vi "Plot legend tester.vi"() -> ()   [LabVIEW 2020]
uses:
  XGrapher.xctl
  Typedefs/Xctrl-ROI type enum.ctl
  Typedefs/Xctl-XY data type definition.ctl
  Typedefs/Xcrtl-Data format definition.ctl
  Typedefs/Xctrl-Data array.ctl
  Data 1.ctl
panel:
  in  "Data In":T1
  out "XY Graph":T6(graph)
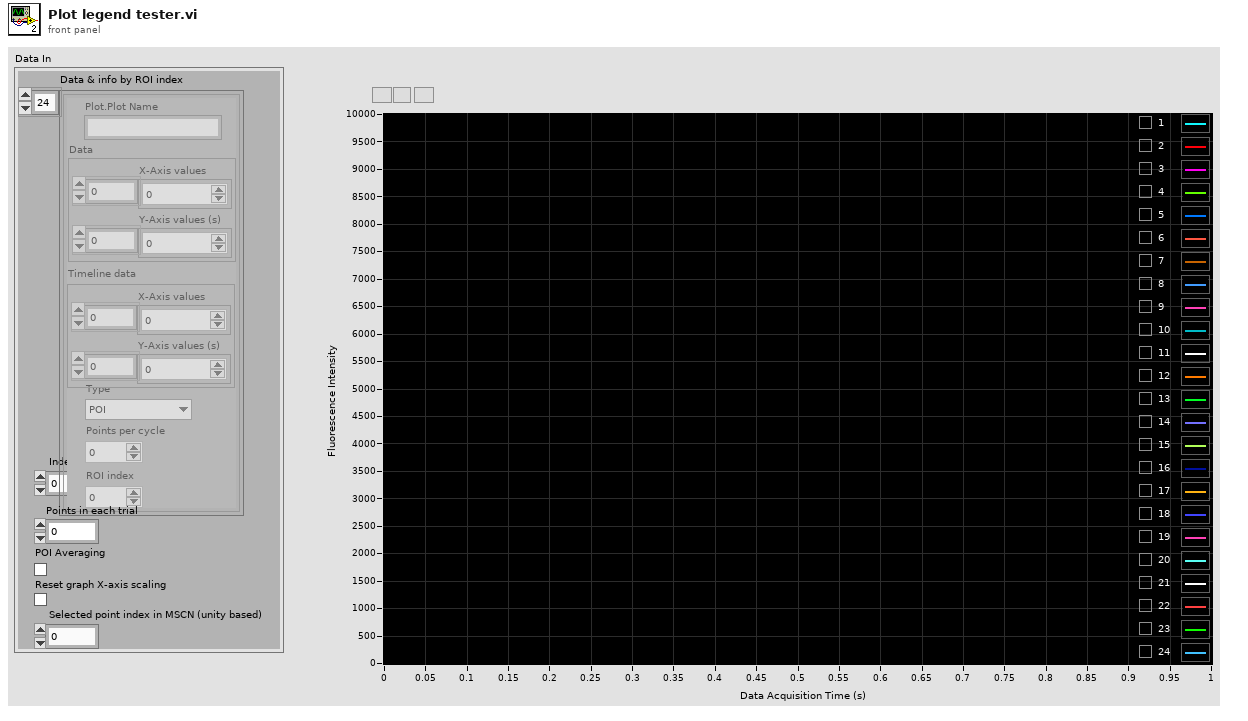
[diagram p1: front panel]
types:
  T1 = typedef "XGrapher.xctl/Data 1.ctl" = cluster{"Data & info by ROI index":T2, "Index of selected plot":u16, "Points in each trial":i32, "POI Averaging":bool, "Reset graph X-axis scaling":bool, "Selected point index in MSCN (unity based)":u16}
  T2 = typedef "Xctrl-Data array.ctl" = T3[]
  T3 = typedef "XGrapher.xctl/Xcrtl-Data format definition.ctl" = cluster{"Plot.Plot Name":string, "Data":T4, "Timeline data":T4, "Type":T5, "Points per cycle":u16, "ROI index":u16}
  T4 = typedef "XGrapher.xctl/Xctl-XY data type definition.ctl" = cluster{"X-Axis values":sgl[], "Y-Axis values (s)":sgl[]}
  T5 = typedef "Xctrl-ROI type enum.ctl" = enum16{"POI", "Mini-scan", "Group"}
  T6 = cluster{"X-Axis values":dbl[], "Y-Axis values":dbl[]}[]
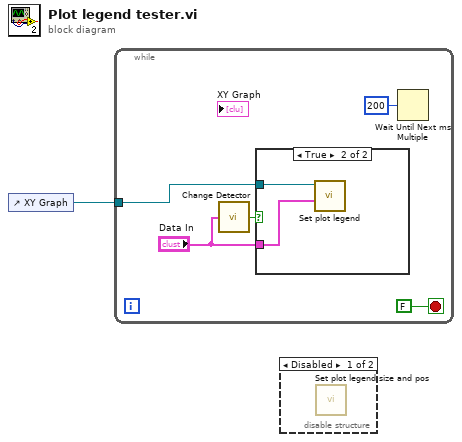
[diagram p0: block diagram]
diagram:
  n1 = control-ref of="XY Graph"() -> (w1:refnum<vi>)
  n2 = while {
    tunnel: w1 -> [w6]
    stop <- FALSE stop-if-true
    n3 = call <userlib>:"Change Detector.vi"("Value"="Data In") -> ("Changed?"=w2:bool)
    n4 = case shown="True" w2 {
      tunnel: w6 -> [_ w8]
      tunnel: "Data In" -> [_ w7]
      frame False {
      }
      frame True {
        n5 = call "Set plot legend.vi"("Data In"=w7, "XYGraph in"=w8) -> ()  [unwired: 8 in, 2 out]
      }
    }
    n6 = Wait Until Next ms Multiple(millisecond multiple=u32 200) -> ()  [unwired: 1 out]
  }
  n7 = disable-structure shown="Disabled" {
    frame Disabled {
      n8 = call "Set plot legend size and pos.vi"() -> ()  [unwired: 11 in, 1 out]
    }
    frame Enabled {
    }
  }
